vi "Theta (SubVI).vi"(8 "error in (no error)":errorcluster, 11 "PWM":dbl) -> (0 "error out":errorcluster, 3 "Theta":dbl)   [LabVIEW 2021]
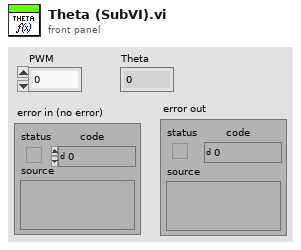
[diagram p1: front panel]
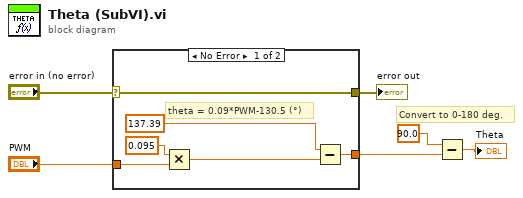
[diagram p0: block diagram]
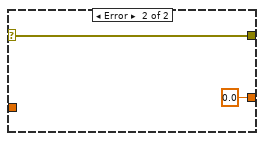
[diagram p2: hidden frame]
diagram:
  # "Convert to 0-180 deg."
  n1 = case shown="No Error" "error in (no error)" {
    selector: "error in (no error)" -> [w7 w14]
    tunnel: [w7 w14] -> w5
    tunnel: "PWM" -> [w9 _]
    tunnel: [w8 0.0] -> w2
    frame No Error {
      # "theta = 0.09*PWM-130.5 (°)"
      n2 = Multiply(x=0.095, y=w9) -> (x*y=w12:dbl)
      n3 = Subtract(x=137.39, y=w12) -> (x-y=w8:dbl)
    }
    frame Error {
    }
  }
  "error out" <- w5
  n4 = Subtract(x=90.0, y=w2) -> (x-y=→"Theta":dbl)
